vi "Autonomous Independent.vi"() -> ()   [LabVIEW 2017]
doc: "This VI is called when autonomous begins, and will automatically be terminated when autonomous ends. You can carry out timed or sensor driven robot movement independently without needing to return to the caller."
uses:
  <vilib>/Rock Robotics/WPI/ThirdParty/Phoenix-LabVIEW/Motor Controller/Controls/CTRE_Phoenix_MotorControl_ControlMode.ctl
  <vilib>/Rock Robotics/WPI/ThirdParty/Phoenix-LabVIEW/Motor Controller/Controls/CTRE_Phoenix_MotorControl_FeedbackDevice.ctl
  Robot Global Data.vi
  <vilib>/Rock Robotics/WPI/ThirdParty/Phoenix-LabVIEW/Motor Controller/Get/CTRE_Phoenix_MotorController_GetSelectedSensorData.vi
panel:
  out "Position (Raw Motor2)":i32
  out "Position (Raw Motor1)":i32
  out "Graph":T1(graph)={"Position (Raw Sensor Units)"=7120, "Position (Raw Sensor Units)"=7133, "Velocity (Raw Sensor Units per 100 ms)"=0, "Velocity (Raw Sensor Units per 100 ms)"=0}
  in  "Max Acceleration 2":i32=300
  in  "Cruise Velocity 2":i32=300
  in  "Distance in native units":dbl=7200.0
  in  "Max Acceleration":i32=300
  in  "Cruise Velocity":i32=300
  # "Be sure to right-click and choose Data Operations>>Make Current Value default if you want to save the array values with the VI"
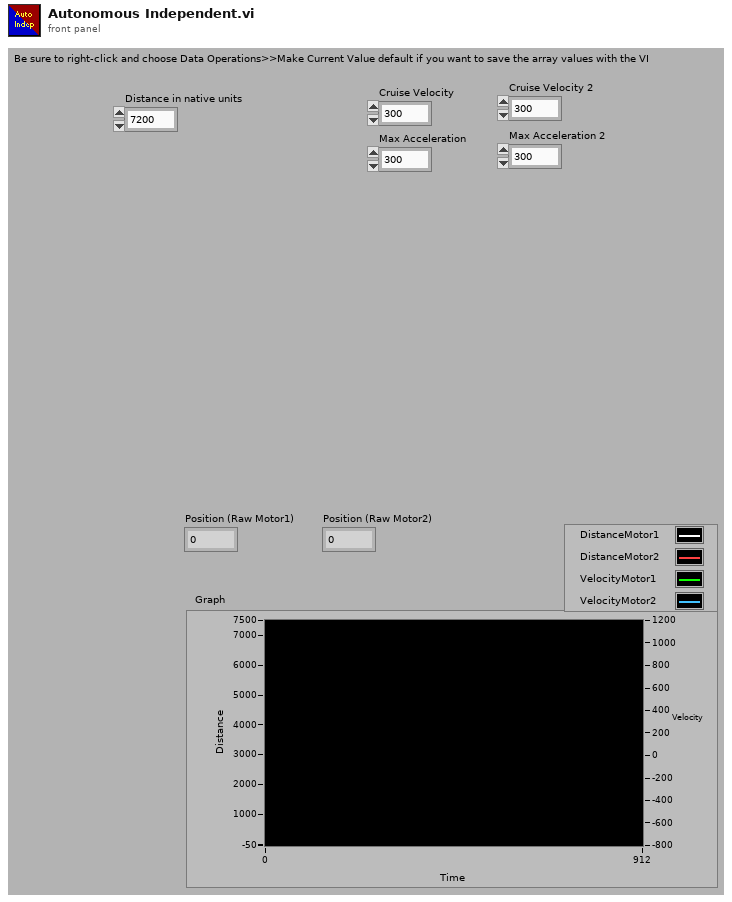
[diagram p1: front panel]
types:
  T1 = cluster{"Position (Raw Sensor Units)":i32, "Position (Raw Sensor Units)":i32, "Velocity (Raw Sensor Units per 100 ms)":i32, "Velocity (Raw Sensor Units per 100 ms)":i32}
  T2 = typedef "WPI_MotorControlDeviceRef.ctl" = cluster{"DeviceStatus":errorcluster, "Type":T3, "PWM":cluster{"PWM Channel":T4, "DeadBand":T5}, "CAN":cluster{"Device Number":u8, "SetOutput VI Ref":variant, "GetOutput VI Ref":variant, "Enable VI Ref":variant, "Disable VI Ref":variant, "Data":variant}, "Invert":bool, "DIO PWM":cluster{"PWM \"Enable\" Channel":T4, "DIOChannel":T6, "PWM Rate":dbl}}
  T3 = typedef "WPI_MotorControlType.ctl" = enum16{"PWM", "CAN", "DIO PWM"}
  T4 = typedef "FPGA_DIOPWMChannel.ctl" = enum8{"PWM 0", "PWM 1", "PWM 2", "PWM 3", "PWM 4", "PWM 5", "PWM 6", "PWM 7", "PWM 8", "PWM 9", "PWM MXP 0", "PWM MXP 1", "PWM MXP 2", "PWM MXP 3", "PWM MXP 4", "PWM MXP 5", "PWM MXP 6", "PWM MXP 7", "PWM MXP 8", "PWM MXP 9", "Invalid"}
  T5 = typedef "WPI_PWMDeadband.ctl" = cluster{"Name":string, "maxPositivePwm":i32, "minPositivePwm":i32, "centerPwm":i32, "maxNegativePwm":i32, "minNegativePwm":i32, "angularRange":u16}
  T6 = typedef "FPGA_DIOChannel.ctl" = enum8{"DIO 0", "DIO 1", "DIO 2", "DIO 3", "DIO 4", "DIO 5", "DIO 6", "DIO 7", "DIO 8", "DIO 9", "DIO MXP 0", "DIO MXP 1", "DIO MXP 2", "DIO MXP 3", "DIO MXP 4", "DIO MXP 5", "DIO MXP 6", "DIO MXP 7", "DIO MXP 8", "DIO MXP 9", "DIO MXP 10", "DIO MXP 11", "DIO MXP 12", "DIO MXP 13", "DIO MXP 14", "DIO MXP 15", "SPI Port CS1", "SPI Port CS2", "SPI Port CS3", "SPI Port MISO", "SPI Port MOSI", "Invalid"}
  T7 = typedef "Auto.ctl" = enum16{"CrossTheLine", "DoNothing"}
  T8 = typedef "RobotPosition.ctl" = enum16{""}
  T9 = typedef "CTRE_Phoenix_MotorControl_ControlMode.ctl" = u16
  T10 = typedef "CTRE_Phoenix_MotorControl_FeedbackDevice.ctl" = i8
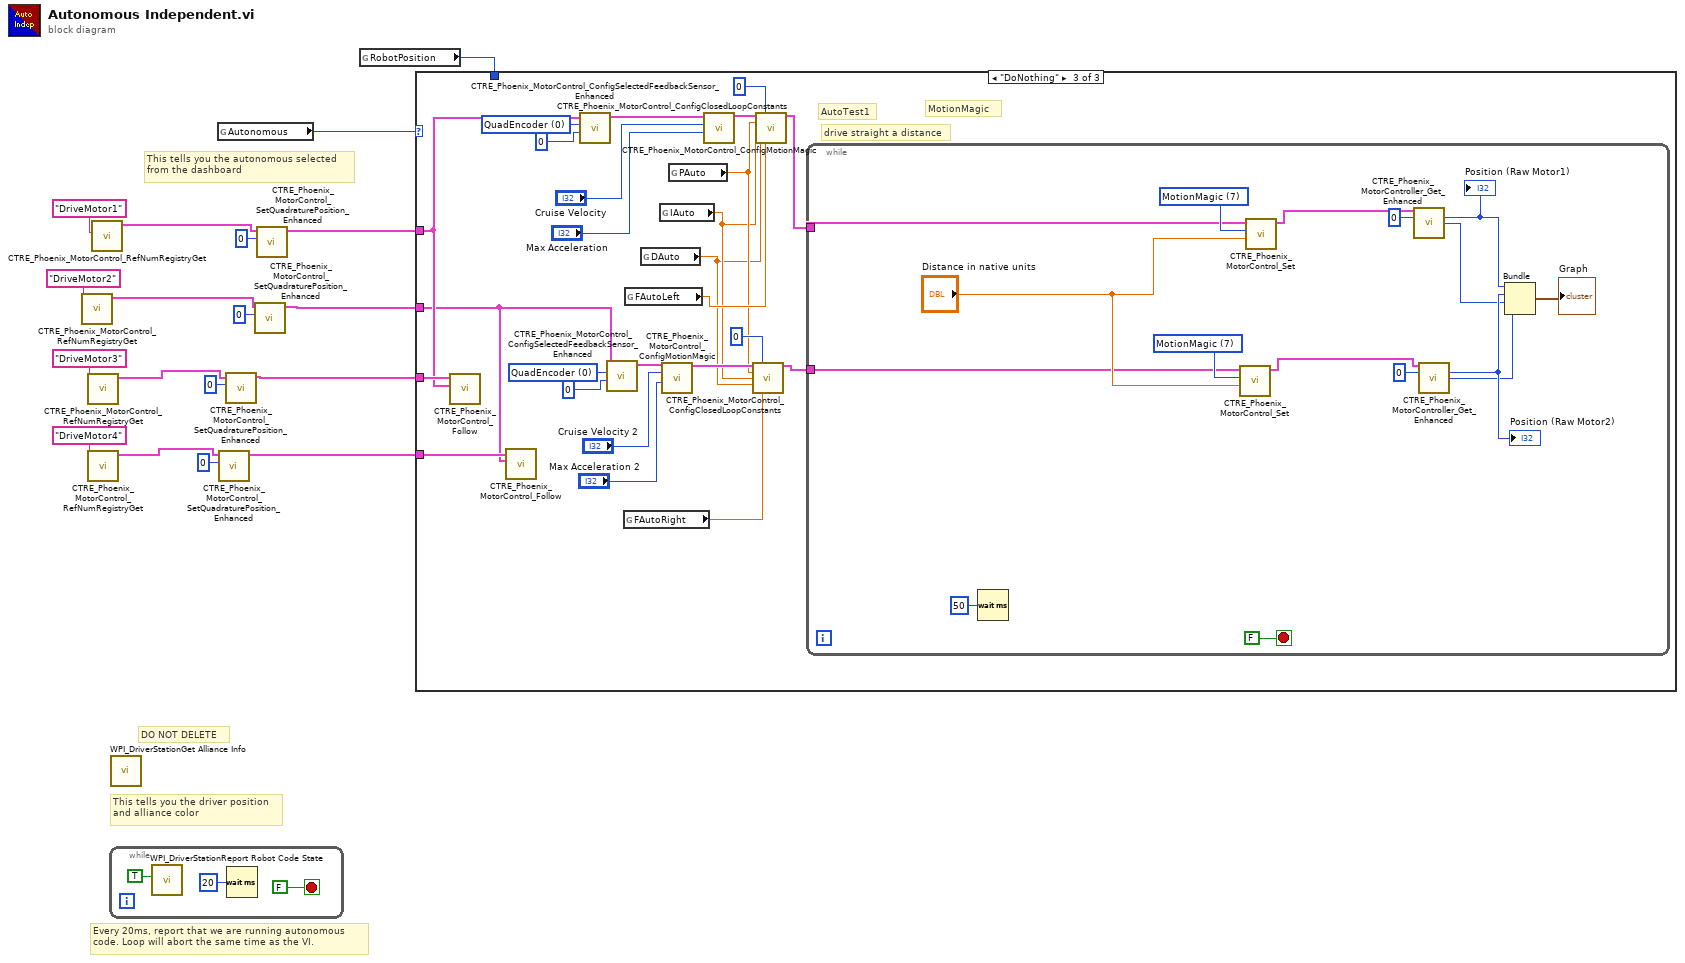
[diagram p0: block diagram]
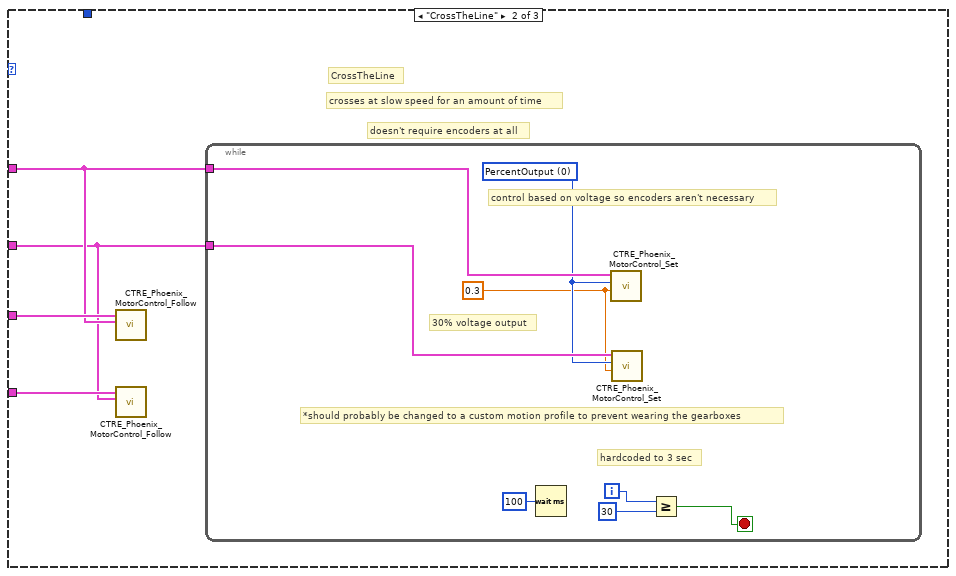
[diagram p3: hidden frame]
diagram:
  # "DO NOT DELETE"
  # "This tells you the autonomous selected\nfrom the dashboard"
  # "Every 20ms, report that we are running autonomous\ncode. Loop will abort the same time as the VI."
  # "This tells you the driver position\nand alliance color"
  n1 = call <vilib>:"CTRE_Phoenix_MotorControl_RefNumRegistryGet.vi"("refnum name"="DriveMotor2") -> ("PhoenixMotorControlDevRef"=w5:T2)  [unwired: 9 in, 1 out]
  n2 = call <vilib>:"CTRE_Phoenix_MotorControl_RefNumRegistryGet.vi"("refnum name"="DriveMotor3") -> ("PhoenixMotorControlDevRef"=w4:T2)  [unwired: 9 in, 1 out]
  n3 = call <vilib>:"CTRE_Phoenix_MotorControl_RefNumRegistryGet.vi"("refnum name"="DriveMotor4") -> ("PhoenixMotorControlDevRef"=w1:T2)  [unwired: 9 in, 1 out]
  n4 = call <vilib>:"CTRE_Phoenix_MotorControl_RefNumRegistryGet.vi"("refnum name"="DriveMotor1") -> ("PhoenixMotorControlDevRef"=w8:T2)  [unwired: 9 in, 1 out]
  n5 = while {
    stop <- FALSE stop-if-true
    n6 = call <vilib>:"WPI_DriverStationReport Robot Code State.vi"("Autonomous"=TRUE) -> ()  [unwired: 10 in, 1 out]
    n7 = Wait (ms)(milliseconds to wait=u32 20) -> ()  [unwired: 1 out]
  }
  n8 = call <vilib>:"WPI_DriverStationGet Alliance Info.vi"() -> ()  [unwired: 12 out]
  n9 = global read "Robot Global Data.vi" "Autonomous"() -> (w18:T7)
  n10 = call <vilib>:"CTRE_Phoenix_MotorControl_SetQuadraturePosition_Enhanced.vi"("New Position"=0, "PhoenixMotorControlDevRef"=w1) -> ("PhoenixMotorControlDevRef"=w2:T2)  [unwired: 8 in, 1 out]
  n11 = call <vilib>:"CTRE_Phoenix_MotorControl_SetQuadraturePosition_Enhanced.vi"("New Position"=0, "PhoenixMotorControlDevRef"=w4) -> ("PhoenixMotorControlDevRef"=w3:T2)  [unwired: 8 in, 1 out]
  n12 = call <vilib>:"CTRE_Phoenix_MotorControl_SetQuadraturePosition_Enhanced.vi"("New Position"=0, "PhoenixMotorControlDevRef"=w5) -> ("PhoenixMotorControlDevRef"=w6:T2)  [unwired: 8 in, 1 out]
  n13 = call <vilib>:"CTRE_Phoenix_MotorControl_SetQuadraturePosition_Enhanced.vi"("New Position"=0, "PhoenixMotorControlDevRef"=w8) -> ("PhoenixMotorControlDevRef"=w7:T2)  [unwired: 8 in, 1 out]
  n14 = global read "Robot Global Data.vi" "RobotPosition"() -> (w17:T8)
  n15 = case shown="\"DoNothing\"" w18 {
    tunnel: w17 -> [_ _ _]
    tunnel: w7 -> [_ w23 w57]
    tunnel: w6 -> [_ w22 w40]
    tunnel: w3 -> [_ w24 w58]
    tunnel: w2 -> [_ w25 w41]
    frame Default {
      # "SWAP W CASE 1 AFTER TESTING IS DONE"
      # "do NOTHING"
      # "DoNothing"
    }
    frame "CrossTheLine" {
      # "doesn't require encoders at all"
      # "crosses at slow speed for an amount of time"
      # "CrossTheLine"
      n16 = call <vilib>:"CTRE_Phoenix_MotorControl_Follow.vi"("Master Controller to Follow"=w23, "PhoenixMotorControlDevRef"=w24) -> ()  [unwired: 8 in, 2 out]
      n17 = call <vilib>:"CTRE_Phoenix_MotorControl_Follow.vi"("Master Controller to Follow"=w22, "PhoenixMotorControlDevRef"=w25) -> ()  [unwired: 8 in, 2 out]
      n18 = while {
        tunnel: w23 -> [w29]
        tunnel: w22 -> [w28]
        i -> [w32]
        stop <- w33 stop-if-true
        w26 = 0.3 ("Output")
        w27 = T9 0 items=["PercentOutput"=0, "Position"=1, "Velocity"=2, "Current"=3, "Follower"=5, "MotionProfile"=6, "MotionMagic"=7, "MotionMagicArc"=8, "MotionProfileArc"=10, "Disabled"=15] ("Control Mode")
        # "*should probably be changed to a custom motion profile to prevent wearing the gearboxes"
        # "control based on voltage so encoders aren't necessary"
        # "30% voltage output"
        # "hardcoded to 3 sec"
        n19 = Wait (ms)(milliseconds to wait=u32 100) -> ()  [unwired: 1 out]
        n20 = call <vilib>:"CTRE_Phoenix_MotorControl_Set.vi"("Output"=w26, "Control Mode"=w27, "PhoenixMotorControlDevRef"=w29) -> ()  [unwired: 7 in, 2 out]
        n21 = call <vilib>:"CTRE_Phoenix_MotorControl_Set.vi"("Output"=w26, "Control Mode"=w27, "PhoenixMotorControlDevRef"=w28) -> ()  [unwired: 7 in, 2 out]
        n22 = Greater Or Equal?(x=w32, y=30) -> (x >= y?=w33:bool)
      }
    }
    frame "DoNothing" {
      w42 = T10 0 items=["None"=-1, "QuadEncoder"=0, "Analog"=2, "Tachometer"=4, "Pulse Width Encoded Position"=8, "Sensor Sum (S0 + S1)"=9, "Sensor Difference (D0 - D1)"=10, "Remote Source 0"=11, "Remote Source 1"=12, "Software Emulated"=15] ("Feedback Device")
      w50 = T10 0 items=["None"=-1, "QuadEncoder"=0, "Analog"=2, "Tachometer"=4, "Pulse Width Encoded Position"=8, "Sensor Sum (S0 + S1)"=9, "Sensor Difference (D0 - D1)"=10, "Remote Source 0"=11, "Remote Source 1"=12, "Software Emulated"=15] ("Feedback Device")
      # "MotionMagic"
      # "drive straight a distance"
      # "AutoTest1"
      n23 = call <vilib>:"CTRE_Phoenix_MotorControl_Follow.vi"("Master Controller to Follow"=w57, "PhoenixMotorControlDevRef"=w58) -> ()  [unwired: 8 in, 2 out]
      n24 = call <vilib>:"CTRE_Phoenix_MotorControl_Follow.vi"("Master Controller to Follow"=w40, "PhoenixMotorControlDevRef"=w41) -> ()  [unwired: 8 in, 2 out]
      n25 = call <vilib>:"CTRE_Phoenix_MotorControl_ConfigSelectedFeedbackSensor_Enhanced.vi"("pidLoopIdx"=0, "Feedback Device"=w50, "PhoenixMotorControlDevRef"=w57) -> ("PhoenixMotorControlDevRef"=w53:T2)  [unwired: 7 in, 1 out]
      n26 = call <vilib>:"CTRE_Phoenix_MotorControl_ConfigSelectedFeedbackSensor_Enhanced.vi"("pidLoopIdx"=0, "Feedback Device"=w42, "PhoenixMotorControlDevRef"=w40) -> ("PhoenixMotorControlDevRef"=w45:T2)  [unwired: 7 in, 1 out]
      n27 = global read "Robot Global Data.vi" "FAutoRight"() -> (w34:dbl)
      n28 = global read "Robot Global Data.vi" "FAutoLeft"() -> (w38:dbl)
      n29 = global read "Robot Global Data.vi" "DAuto"() -> (w35:dbl)
      n30 = global read "Robot Global Data.vi" "IAuto"() -> (w36:dbl)
      n31 = call <vilib>:"CTRE_Phoenix_MotorControl_ConfigMotionMagic.vi"("Acceleration"="Max Acceleration 2", "Cruise Velocity"="Cruise Velocity 2", "PhoenixMotorControlDevRef"=w45) -> ("PhoenixMotorControlDevRef"=w48:T2)  [unwired: 7 in, 1 out]
      n32 = global read "Robot Global Data.vi" "PAuto"() -> (w37:dbl)
      n33 = call <vilib>:"CTRE_Phoenix_MotorControl_ConfigMotionMagic.vi"("Acceleration"="Max Acceleration", "Cruise Velocity"="Cruise Velocity", "PhoenixMotorControlDevRef"=w53) -> ("PhoenixMotorControlDevRef"=w56:T2)  [unwired: 7 in, 1 out]
      n34 = call <vilib>:"CTRE_Phoenix_MotorControl_ConfigClosedLoopConstants.vi"("PhoenixMotorControlDevRef"=w48, "slotIdx"=0, "P"=w37, "I"=w36, "D"=w35, "F"=w34) -> ("PhoenixMotorControlDevRef"=w39:T2)  [unwired: 8 in, 1 out]
      n35 = call <vilib>:"CTRE_Phoenix_MotorControl_ConfigClosedLoopConstants.vi"("PhoenixMotorControlDevRef"=w56, "slotIdx"=0, "P"=w37, "I"=w36, "D"=w35, "F"=w38) -> ("PhoenixMotorControlDevRef"=w49:T2)  [unwired: 8 in, 1 out]
      n36 = while {
        tunnel: w49 -> [w71]
        tunnel: w39 -> [w68]
        stop <- FALSE stop-if-true
        w70 = T9 7 items=["PercentOutput"=0, "Position"=1, "Velocity"=2, "Follower"=5, "MotionProfile"=6, "MotionMagic"=7, "MotionMagicArc"=8, "TimedPercentOutput"=9, "Disabled"=15] ("Control Mode")
        w74 = T9 7 items=["PercentOutput"=0, "Position"=1, "Velocity"=2, "Follower"=5, "MotionProfile"=6, "MotionMagic"=7, "MotionMagicArc"=8, "TimedPercentOutput"=9, "Disabled"=15] ("Control Mode")
        n37 = Wait (ms)(milliseconds to wait=u32 50) -> ()  [unwired: 1 out]
        n38 = call <vilib>:"CTRE_Phoenix_MotorControl_Set.vi"("Output"="Distance in native units", "Control Mode"=w70, "PhoenixMotorControlDevRef"=w68) -> ("PhoenixMotorControlDevRef"=w64:T2)  [unwired: 7 in, 1 out]
        n39 = call <vilib>:"CTRE_Phoenix_MotorControl_Set.vi"("Output"="Distance in native units", "Control Mode"=w74, "PhoenixMotorControlDevRef"=w71) -> ("PhoenixMotorControlDevRef"=w66:T2)  [unwired: 7 in, 1 out]
        n40 = call-poly <vilib>:"CTRE_Phoenix_MotorController_Get_Enhanced.vi"("PhoenixMotorControlDevRef"=w66, "pidLoopIdx"=u32 0) -> ("Position (Raw Sensor Units)"=w63:i32, "Velocity (Raw Sensor Units per 100 ms)"=w61:i32)  [unwired: 10 in, 2 out]
        "Position (Raw Motor1)" <- w63
        n41 = call-poly <vilib>:"CTRE_Phoenix_MotorController_Get_Enhanced.vi"("PhoenixMotorControlDevRef"=w64, "pidLoopIdx"=u32 0) -> ("Position (Raw Sensor Units)"=w62:i32, "Velocity (Raw Sensor Units per 100 ms)"=w60:i32)  [unwired: 10 in, 2 out]
        "Position (Raw Motor2)" <- w62
        n42 = Bundle("Position (Raw Sensor Units)"=w63, "Position (Raw Sensor Units)"=w62, "Velocity (Raw Sensor Units per 100 ms)"=w61, "Velocity (Raw Sensor Units per 100 ms)"=w60) -> (→"Graph":T1)  [unwired: 1 in]
      }
    }
  }
